vi "Read Control Refnum.vi"(11 "TerminalReferenceBinding in":refnum<class "TerminalPropertyBinding.lvclass">) -> (2 "Ctl Refnum":refnum<vi>, 3 "TerminalReferenceBinding out":refnum<class "TerminalPropertyBinding.lvclass">)   [LabVIEW 2020, in "MVA Framework.lvlib" / "TerminalPropertyBinding.lvclass"]
doc: "读取控件引用"
uses:
  TerminalPropertyBinding.lvclass
  TerminalPropertyBinding.lvclass/TerminalPropertyBinding.ctl
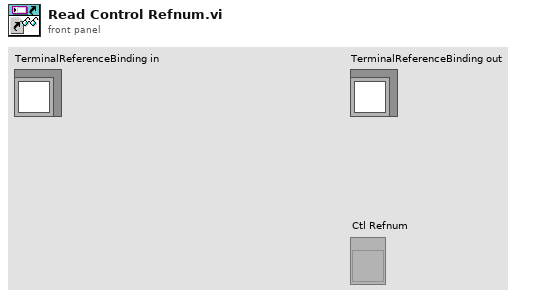
[diagram p1: front panel]
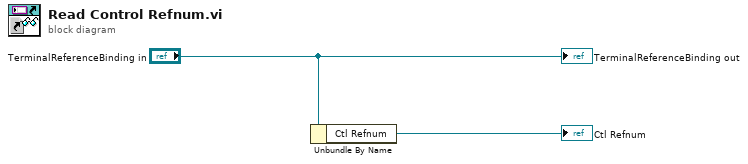
[diagram p0: block diagram]
diagram:
  n1 = Unbundle By Name("TerminalReferenceBinding in") -> ("Ctl Refnum"=→"Ctl Refnum":refnum<vi>)
  "TerminalReferenceBinding out" <- "TerminalReferenceBinding in"
